vi "Generation.vi"(8 "error in (no error)":errorcluster, 11 "Configuration in":refnum<class "Configuration.lvclass">) -> (0 "error out":errorcluster, 3 "Configuration out":refnum<class "Configuration.lvclass">)   [LabVIEW 2026, in "Hardware.lvlib" / "HW with output config.lvclass"]
uses:
  HW with output config.lvclass
  configuration/Configuration.lvclass
  C:/Users/E2013170/Documents/GitHub/Measurement-Utility-Reference/source/configuration/Configuration.lvclass
  C:/Users/E2013170/Documents/GitHub/Measurement-Utility-Reference/source/framework/Hardware/HW Config/HW Configuration.lvclass
  HW Configuration.lvclass/HW Configuration.ctl
  HW with output config.lvclass/HW with output config.ctl
  HW Configuration.lvclass
panel:
  in  "remove as output":bool
  out "Output Channels":string[](array[string])
  in  "add as output":bool
  in  "Enable Generation":bool
  in  "Select IO Channel":u16(ring)
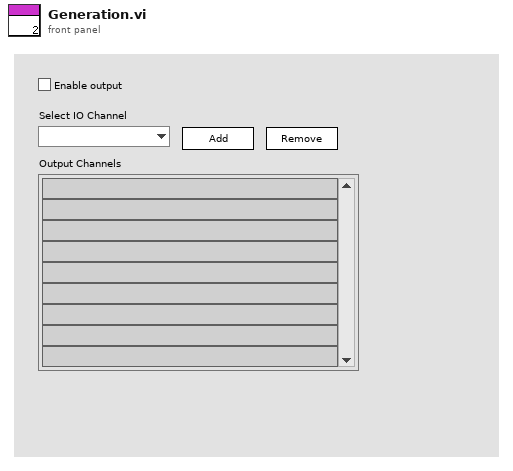
[diagram p1: front panel]
types:
  T1 = enum8{"Enabled", "Disabled", "Disabled and Grayed Out"}
  T2 = cluster{"Device Name":string, "Channel Mapping (Device -> Channel)":string[][]}
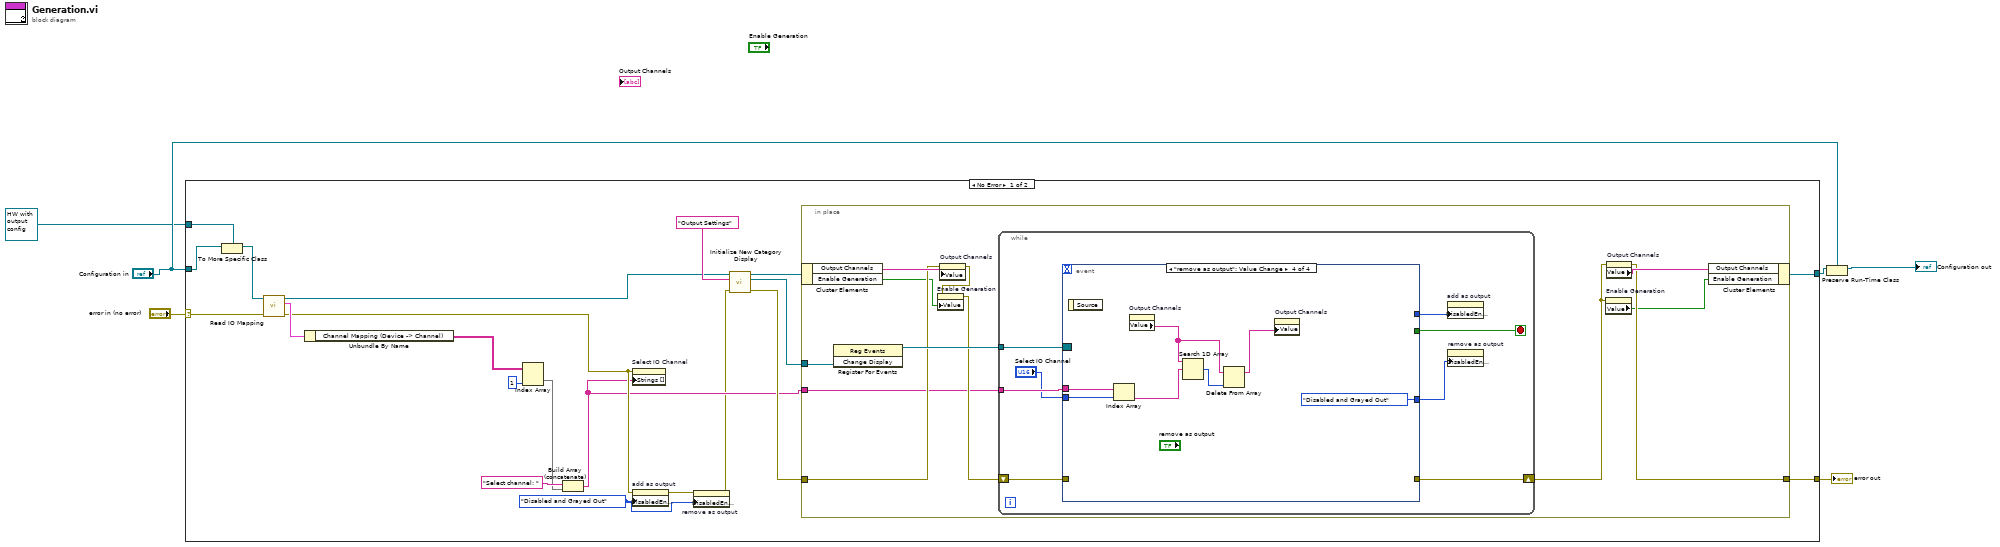
[diagram p0: block diagram]
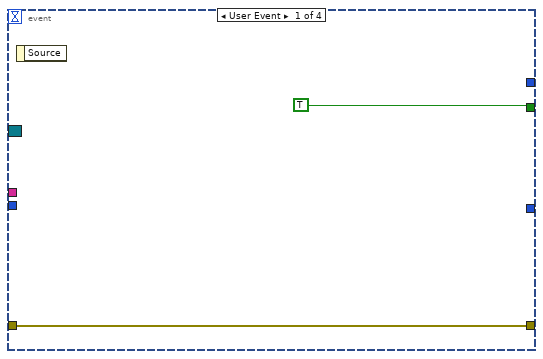
[diagram p2: hidden frame]
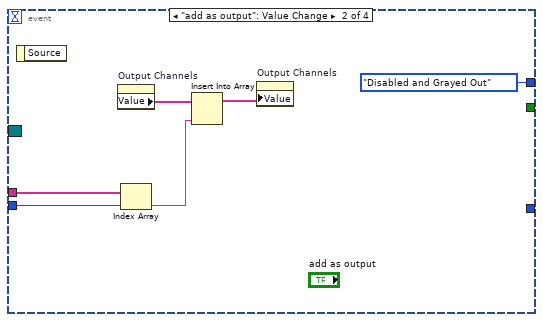
[diagram p3: hidden frame]
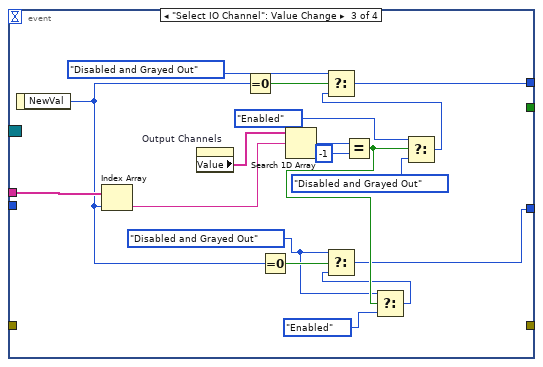
[diagram p4: hidden frame]
diagram:
  n1 = case shown="No Error" "error in (no error)" {
    selector: "error in (no error)" -> [w18 w82]
    tunnel: [w21 w81] -> w3
    tunnel: [w20 w82] -> w6
    tunnel: "Configuration in" -> [w24 w81]
    tunnel: refnum<class "HW with output config.lvclass"> refnum ("Hardware.lvlib:HW with output config.lvclass") -> [w23 _]
    frame No Error {
      w9 = T1."Disabled and Grayed Out" ("Disabled")
      n2 = To More Specific Class(target class=w23, reference=w24) -> (specific class reference=w19:refnum<class "HW with output config.lvclass">)  [unwired: 1 in, 1 out]
      n3 = call "Read IO Mapping.vi"("error in (no error)"=w18, "HW Configuration in"=w19) -> ("error out"=w12:errorcluster, "IO Mapping"=w16:T2, "HW Configuration out"=w17:refnum<class "HW with output config.lvclass">)  [unwired: 7 in]
      n4 = Unbundle By Name(w16) -> ("Channel Mapping (Device -> Channel)"=w15:string[][])
      n5 = Index Array(array=w15, index (col)=1 ("disabled index (col)")) -> (element=w11:string[])  [unwired: 1 in]
      n6 = Build Array (concatenate)("Select channel: " ("Name to Display"), w11) -> (w10:string[])
      n7 = property on="Select IO Channel" class="Ring (strict)"(error in=w12, "Strings []"=w10) -> ()  [unwired: 1 in, 2 out]
      n8 = property on="add as output" class="Bool"(error in=w12, "DisabledEnum"=w9) -> (error out=w8:errorcluster)  [unwired: 1 in, 1 out]
      n9 = property on="remove as output" class="Bool"(error in=w8, "DisabledEnum"=w9) -> (error out=w7:errorcluster)  [unwired: 1 in, 1 out]
      n10 = call "Initialize New Category Display.vi"("error in (no error)"=w7, "Name to Display"="Output Settings", "Configuration in"=w17) -> ("error out"=w26:errorcluster, "Change Display"=w27:refnum<user-event>, "Configuration Out"=w22:refnum<class "HW with output config.lvclass">)  [unwired: 6 in]
      n11 = in-place {
        in-place-border: w27 -> [w39]
        in-place-border: w26 -> [w36]
        in-place-border: [w34] -> w20
        in-place-border: w10 -> [w28]
        n12 = in-place-cluster #1(w22) -> ("Output Channels"=w37:string[], "Enable Generation"=w33:bool)
        n13 = register-events(w39) -> (reference out=w38:refnum<event-registration>)  [unwired: 2 in, 1 out]
        n14 = property on="Output Channels" class="Arr (strict)"(error in=w36, "Value"=w37) -> (error out=w32:errorcluster)  [unwired: 1 in, 1 out]
        n15 = property on="Enable Generation" class="Bool (strict)"(error in=w32, "Value"=w33) -> (error out=w31:errorcluster)  [unwired: 1 in, 1 out]
        n16 = while {
          tunnel: w38 -> [w46]
          shift-right: [w45] -> w30
          shift-left: w31 -> [w44]
          tunnel: w28 -> [w43]
          stop <- w47 stop-if-true
          n17 = event shown="[3] \"remove as output\": Value Change" {
            selector: w46 -> [_ _ _ _]
            dyn-events: _ -> [_ _ _ _]
            timeout: _ -> [_ _ _ _]
            tunnel: [TRUE _ _ _] -> w47
            tunnel: [w48 _ _ _] -> w45
            tunnel: w44 -> [w48 _ _ _]
            tunnel: w43 -> [_ w55 w71 w80]
            tunnel: [_ T1."Disabled and Grayed Out" ("Disabled") w64 _] -> w42
            tunnel: [_ _ w56 T1."Disabled and Grayed Out" ("Disabled")] -> w41
            tunnel: "Select IO Channel" -> [_ w51 _ w79]
            event User Event {
              n18 = event-data() -> ()  [unwired: 1 in, 1 out]
            }
            event "add as output": Value Change {
              n19 = event-data() -> ()  [unwired: 1 in, 1 out]
              n20 = property on="Output Channels" class="Arr (strict)"() -> ("Value"=w54:string[])  [unwired: 2 in, 2 out]
              n21 = Index Array(array=w55, index=w51) -> (element=w53:string)
              n22 = Insert Into Array(array=w54, new element=w53) -> (w52:string[])  [unwired: 1 in]
              n23 = property on="Output Channels" class="Arr (strict)"("Value"=w52) -> ()  [unwired: 2 in, 2 out]
            }
            event "Select IO Channel": Value Change {
              w57 = T1."Disabled and Grayed Out" ("Disabled")
              n24 = event-data() -> ("NewVal"=w62:u16)  [unwired: 1 in]
              n25 = Index Array(array=w71, index=w62) -> (element=w70:string)
              n26 = property on="Output Channels" class="Arr (strict)"() -> ("Value"=w72:string[])  [unwired: 2 in, 2 out]
              n27 = Equal To 0?(x=w62) -> (x = 0?=w73:bool)
              n28 = Equal To 0?(x=w62) -> (x = 0?=w61:bool)
              n29 = Search 1D Array(1D array=w72, element=w70) -> (index of element=w69:i32)  [unwired: 1 in]
              n30 = Equal?(x=w69, y=-1) -> (x = y?=w60:bool)
              n31 = Select(t=w57, s=w60, f=T1."Enabled" ("Disabled")) -> (s? t:f=w58:T1)
              n32 = Select(t=w57, s=w61, f=w58) -> (s? t:f=w56:T1)
              n33 = Select(t=T1."Enabled" ("Disabled"), s=w60, f=T1."Disabled and Grayed Out" ("Disabled")) -> (s? t:f=w65:T1)
              n34 = Select(t=T1."Disabled and Grayed Out" ("Disabled"), s=w73, f=w65) -> (s? t:f=w64:T1)
            }
            event "remove as output": Value Change {
              n35 = event-data() -> ()  [unwired: 1 in, 1 out]
              n36 = Index Array(array=w80, index=w79) -> (element=w78:string)
              n37 = property on="Output Channels" class="Arr (strict)"() -> ("Value"=w77:string[])  [unwired: 2 in, 2 out]
              n38 = Search 1D Array(1D array=w77, element=w78) -> (index of element=w76:i32)  [unwired: 1 in]
              n39 = Delete From Array(array=w77, index=w76) -> (array with subset deleted=w75:string[])  [unwired: 1 in, 1 out]
              n40 = property on="Output Channels" class="Arr (strict)"("Value"=w75) -> ()  [unwired: 2 in, 2 out]
            }
          }
          n41 = property on="add as output" class="Bool"("DisabledEnum"=w42) -> ()  [unwired: 2 in, 2 out]
          n42 = property on="remove as output" class="Bool"("DisabledEnum"=w41) -> ()  [unwired: 2 in, 2 out]
        }
        n43 = property on="Enable Generation" class="Bool (strict)"(error in=w30) -> ("Value"=w29:bool)  [unwired: 1 in, 2 out]
        n44 = property on="Output Channels" class="Arr (strict)"(error in=w30) -> (error out=w34:errorcluster, "Value"=w35:string[])  [unwired: 1 in, 1 out]
        n45 = in-place-cluster #1("Output Channels"=w35, "Enable Generation"=w29) -> (w21:refnum<class "HW with output config.lvclass">)
      }
    }
    frame Error {
    }
  }
  "error out" <- w6
  n46 = Preserve Run-Time Class(object in=w3, 2:"Configuration in") -> (object out=→"Configuration out":refnum<class "Configuration.lvclass">)  [unwired: 1 in, 1 out]
